vi "updateModelNumber.vi"(8 "Error In":errorcluster, 9 "Modal Name":string, 10 "Model Number":i32, 11 "DB File Path":path) -> (0 "Error Out":errorcluster)   [LabVIEW 2018]
panel:
  out "String":string
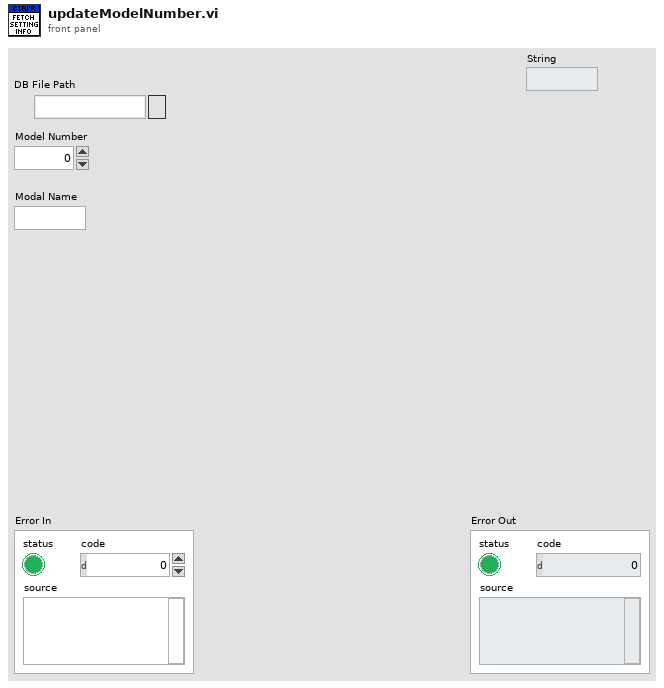
[diagram p1: front panel]
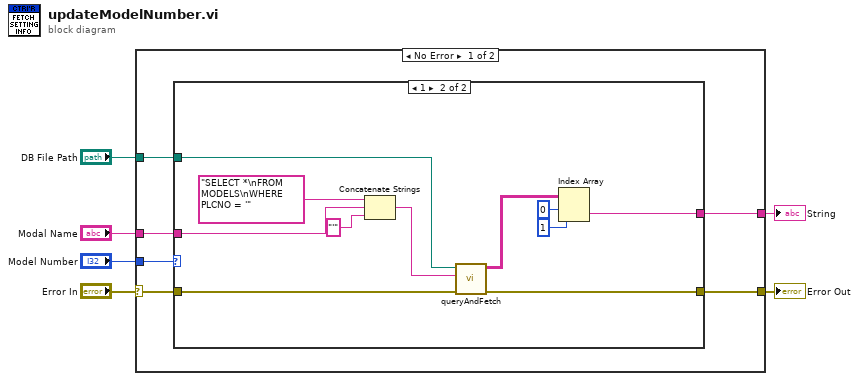
[diagram p0: block diagram]
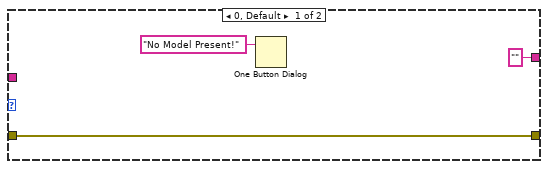
[diagram p2: hidden frame]
diagram:
  n1 = case shown="No Error" "Error In" {
    selector: "Error In" -> [w11 w27]
    tunnel: "Model Number" -> [w12 _]
    tunnel: [w10 w27] -> w4
    tunnel: "DB File Path" -> [w9 _]
    tunnel: [w8 _] -> w1
    tunnel: "Modal Name" -> [w7 _]
    frame No Error {
      n2 = case shown="1" w12 {
        tunnel: w11 -> [w15 w26]
        tunnel: [w15 w25] -> w10
        tunnel: w9 -> [_ w24]
        tunnel: ["" ("String") w18] -> w8
        tunnel: w7 -> [_ w16]
        frame 0, Default {
          n3 = One Button Dialog(message="No Model Present!") -> ()  [unwired: 1 in, 1 out]
        }
        frame 1 {
          n4 = Concatenate Strings("SELECT *\nFROM MODELS\nWHERE PLCNO = '" ("Query"), w16, "'" ("string")) -> (w17:string)
          n5 = call "queryAndFetch.vi"("Error In"=w26, "Query"=w17, "DB File Path"=w24) -> ("Error Out"=w25:errorcluster, "Result Table"=w21:string[][])  [unwired: 7 in]
          n6 = Index Array(array=w21, index (row)=0, index (col)=1 ("disabled index (col)")) -> (element=w18:string)
        }
      }
    }
    frame Error {
    }
  }
  "Error Out" <- w4
  "String" <- w1
